vi "Get Power Meter Default Value.vi"(0 "SG Path PM Accessor in":refnum<class "SG Path PM Accessor Base.lvclass">, 11 "error in (no error)":errorcluster) -> (4 "SG Path PM Accessor out":refnum<class "SG Path PM Accessor Base.lvclass">, 6 "Power Meter out":refnum<class "Power Meter Base.lvclass">, 15 "error out":errorcluster)   [LabVIEW 2023, in "RFFixtureCharact.Instruments.lvlib" / "SG Path PM Accessor Base.lvclass"]
uses:
  SG Path PM Accessor Base.lvclass
  Power Meter Base/Power Meter Base.lvclass
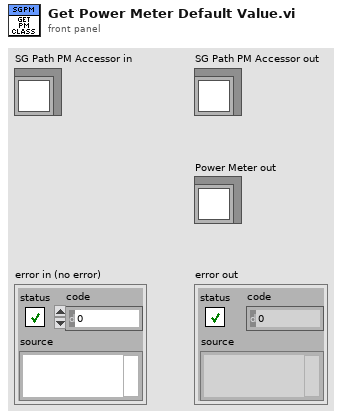
[diagram p1: front panel]
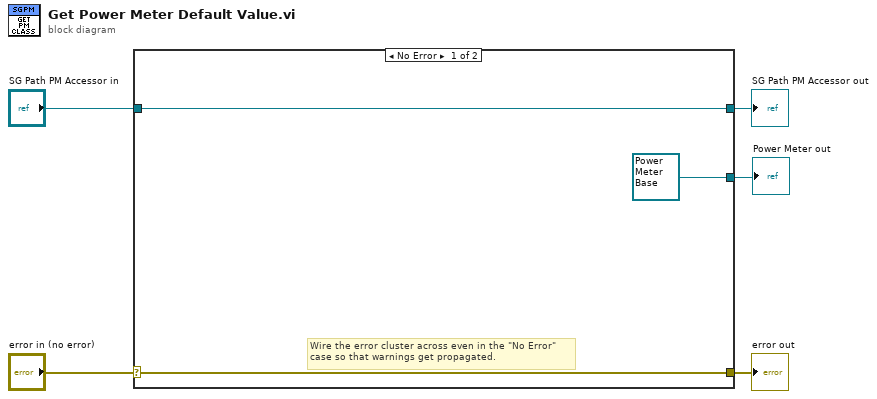
[diagram p0: block diagram]
diagram:
  n1 = case shown="No Error" "error in (no error)" {
    selector: "error in (no error)" -> [w7 w10]
    tunnel: [w7 w10] -> w4
    tunnel: [w8 w9] -> w2
    tunnel: "SG Path PM Accessor in" -> [w8 w9]
    tunnel: [refnum<class "Power Meter Base.lvclass"> refnum ("STS Scalar Fixture Charact.lvlib:Power Meter Base.lvclass") _] -> w1
    frame No Error {
      # "Wire the error cluster across even in the \"No Error\"\ncase so that warnings get propagated."
    }
    frame Error {
    }
  }
  "error out" <- w4
  "SG Path PM Accessor out" <- w2
  "Power Meter out" <- w1
